vi "Save.vi"(8 "error in (no error)":errorcluster, 9 "Prompt":bool=TRUE, 10 "Save_As":bool, 11 "reference in":refnum<class "Object_Editor.lvclass">) -> (0 "error out":errorcluster, 3 "reference out":refnum<class "Object_Editor.lvclass">)   [LabVIEW 2022 SP3, in "Object_Editor.lvlib" / "Object_Editor.lvclass"]
uses:
  Object_Editor.lvclass
  Components/ViPER.lvlibp/ViPER.lvclass
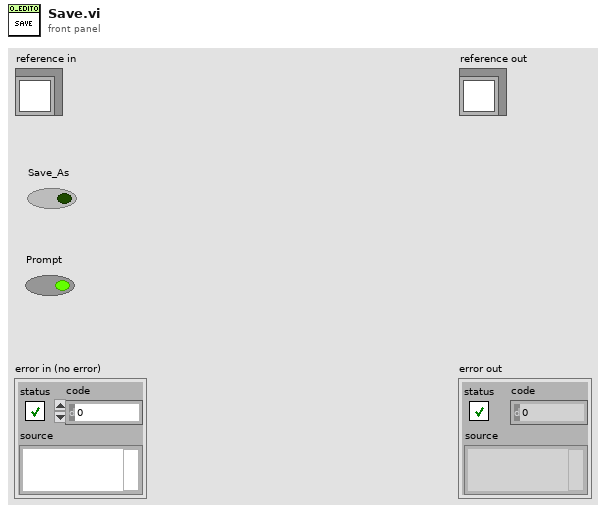
[diagram p1: front panel]
types:
  T1 = typedef "Object_Editor.lvlib/Object_Editor.lvclass/ObjectAttributes.ctl" = cluster{"Config":T2, "Tree":refnum<vi>, "Mod_Bit":bool, "File_Path":path, "Object":refnum<class "ViPER.lvclass">}
  T2 = typedef "Object_Editor.lvlib/Object_Editor.lvclass/Config.ctl" = cluster{"default":string}
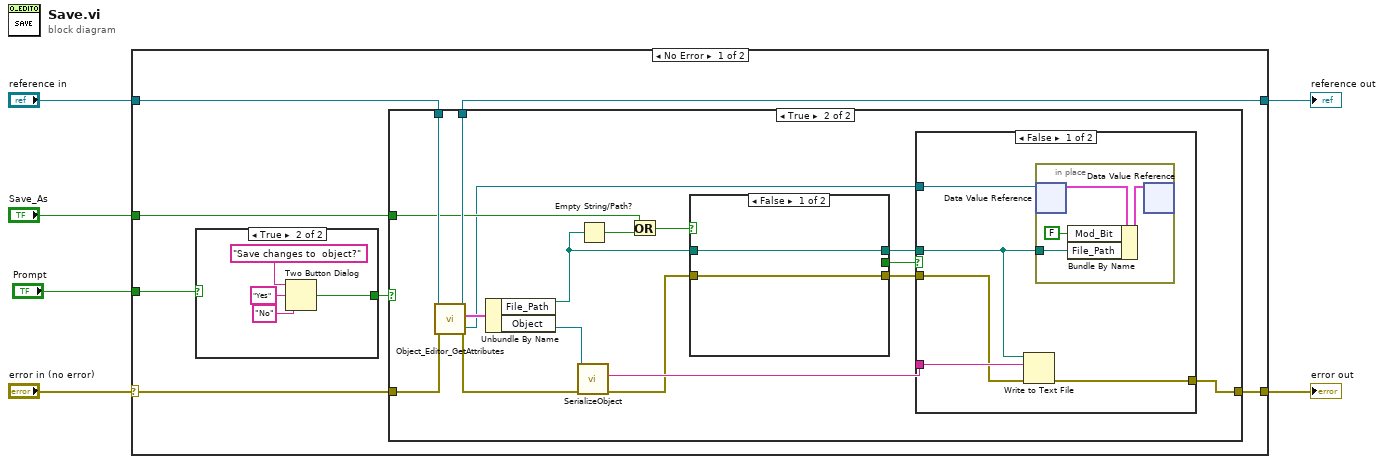
[diagram p0: block diagram]
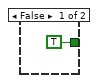
[diagram p2: hidden frame]
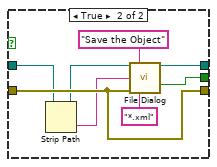
[diagram p5: hidden frame]
diagram:
  n1 = case shown="No Error" "error in (no error)" {
    selector: "error in (no error)" -> [w13 w59]
    tunnel: [w10 w59] -> w5
    tunnel: [w11 w58] -> w3
    tunnel: "reference in" -> [w12 w58]
    tunnel: "Save_As" -> [w9 _]
    tunnel: "Prompt" -> [w7 _]
    frame No Error {
      n2 = case shown="True" w7 {
        tunnel: [TRUE ("T button?") w17] -> w8
        frame False {
        }
        frame True {
          n3 = Two Button Dialog(message="Save changes to  object?", 1:"No" ("F button name (\"Cancel\")"), 2:"Yes" ("T button name (\"OK\")")) -> (T button?=w17:bool)
        }
      }
      n4 = case shown="True" w8 {
        tunnel: w13 -> [w19 w37]
        tunnel: w12 -> [w20 w36]
        tunnel: [w20 w35] -> w11
        tunnel: [w19 w31] -> w10
        tunnel: w9 -> [_ w25]
        frame False {
        }
        frame True {
          n5 = call "Object_Editor_GetAttributes.vi"("error in (no error)"=w37, "reference in"=w36) -> ("error out"=w32:errorcluster, "DataRef"=w21:refnum<data-value>, "Data"=w34:T1, "reference out"=w35:refnum<class "Object_Editor.lvclass">)  [unwired: 6 in]
          n6 = Unbundle By Name(w34) -> ("File_Path"=w26:path, "Object"=w33:refnum<class "ViPER.lvclass">)
          n7 = call-dynamic "SerializeObject.vi"("error in (no error)"=w32, "ViPER_Base in"=w33) -> ("error out"=w29:errorcluster, "Object XML"=w30:string)  [unwired: 7 in, 1 out]
          n8 = Empty String/Path?(string/path=w26) -> (empty?=w24:bool)
          n9 = Or(x=w25, y=w24) -> (x .or. y?=w23:bool)
          n10 = case shown="False" w23 {
            tunnel: w29 -> [w49 w54]
            tunnel: [w49 w54] -> w28
            tunnel: w26 -> [w48 w52]
            tunnel: [w48 w56] -> w27
            tunnel: [_ w55] -> w22
            frame False {
            }
            frame True {
              n11 = Strip Path(path=w52) -> (stripped path=w51:path, name=w50:string)
              n12 = call "File Dialog"("start path"=w51, "prompt"="Save the Object", "default name"=w50, "error in"=w54, "pattern (all files)"="*.xml") -> ("selected path"=w56:path, "cancelled"=w55:bool)  [unwired: 7 in, 2 out]
            }
          }
          n13 = case shown="False" w22 {
            tunnel: [w42 w47] -> w31
            tunnel: w30 -> [w41 _]
            tunnel: w28 -> [w40 w47]
            tunnel: w27 -> [w38 _]
            tunnel: w21 -> [w39 _]
            frame False {
              n14 = Write to Text File(file (use dialog)=w38, text=w41, error in=w40) -> (error out=w42:errorcluster)  [unwired: 1 in, 2 out]
              n15 = in-place {
                in-place-border: w38 -> [w43]
                n16 = in-place-dvr #1(w39) -> (w46:T1)  [unwired: 1 out]
                n17 = Bundle By Name(cluster=w46, "Mod_Bit"=FALSE, "File_Path"=w43) -> (w45:T1)
                n18 = in-place-dvr #1(w45) -> ()  [unwired: 2 out]
              }
            }
            frame True {
            }
          }
        }
      }
    }
    frame Error {
    }
  }
  "error out" <- w5
  "reference out" <- w3
